vi "Stop Stream VI.vi"(8 "error in (no error)":errorcluster, 11 "Filter_Wheel in":refnum<class "Filter_Wheel.lvclass">) -> (0 "error out":errorcluster, 3 "Filter_Wheel out":refnum<class "Filter_Wheel.lvclass">)   [LabVIEW 2018, in "Filter_Wheel.lvclass"]
uses:
  Filter_Wheel.lvclass
  Filter_Wheel.lvclass/Filter_Wheel.ctl
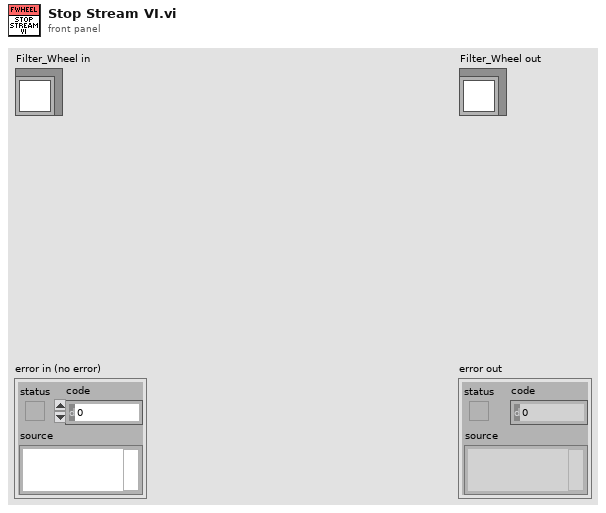
[diagram p1: front panel]
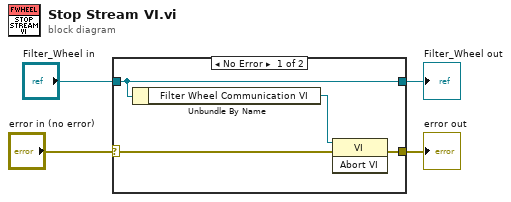
[diagram p0: block diagram]
diagram:
  n1 = case shown="No Error" "error in (no error)" {
    selector: "error in (no error)" -> [w8 w10]
    tunnel: [w7 w10] -> w3
    tunnel: [w6 w9] -> w1
    tunnel: "Filter_Wheel in" -> [w6 w9]
    frame No Error {
      n2 = Unbundle By Name(w6) -> ("Filter Wheel Communication VI"=w5:refnum<vi>)
      n3 = invoke class="VI" method="Abort VI"(reference=w5, error in=w8) -> (error out=w7:errorcluster)  [unwired: 1 in, 2 out]
    }
    frame Error {
    }
  }
  "error out" <- w3
  "Filter_Wheel out" <- w1
